vi "App - RUS scan V1.vi"(0 "Lock-in DAQ settings":T9={"Lockin mode"=enum."NI-DAQ", "DAQmx Device"="Dev2", "SR Lockin"="GPIB0::10::INSTR", "Clock Multiplier"=64, "Low-pass filter"=enum."No filtering", "Ranges and couplings "=[{"Range"=2.5, "Coupling"=10106}], "Samples per read"=20, "Record IF"=FALSE, "Auto-phase"=FALSE} {"Ranges and couplings"."Coupling" items=["default"=-1, "RSE"=10083, "NRSE"=10078, "Differential"=10106, "Pseudodifferential"=12529]}, 1 "Save data settings":T10={"Save data"=TRUE, "Data Root Path"=path "E:/data/Ultrasound/Experiment/ProbeTest/Birdcage/YBCO_6_opt/1_test", "File Prefix"="300.05900K_100_3500_2.00000V_0.65333T_Jul07-2013__19-17-53_", "File Format"=enum."BINARY", "Save column names"=FALSE, "File Comments"="\r\nColumns:Frequency\\tX\\tY\r\n    ITC Temp= 299.200000\r\n    LTC Temp= 0.000000\r\n          ITC_set=295.00000\r\n", "User/Prj"="<User Name/Project Description>"}, 5 "temperature":dbl=300.059, 7 "sweep settings":T6={"wait between \nsweeps (min) "=0.0, "Bypass error dialog"=TRUE, "time in gamma PID?"=FALSE, "power PID?"=FALSE, "range factor"=1.05, "min gamma(kHz)"=0.002, "max step(Hz)"=3000.0, "min step(Hz)"=0.002, "save freq units"=enum."kHz", "Zero amplitude\nat the end"=FALSE, "time in Gamma --OK"=FALSE, "scan mode"=enum."uniform", "power mode "=enum."power vs Temp"}, 9 "Fast swep settings":T8={"Update rate (Hz)"=500.0, "Start F, Hz"=100000.0, "Stop F"=3500000.0, "Number of points"=225000, "Amplitude"=2.0, "Init&amplitude"=TRUE, "IF"=1000.0, "Time constant"=0.001} {"IF" format="%#_6p"; "Amplitude" min=0.0 max=2.5; "Number of points" format="%.0p"; "Stop F" format="%#_6p"; "Start F, Hz" format="%#_6p"; "Update rate (Hz)" format="%0.2f"}, 11 "error in (no error)":errorcluster) -> (6 "Actual file path":path=path "E:/data/Ultrasound/Experiment/ProbeTest/Birdcage/YBCO_6_opt/1_test/July_2013/070713/300.06500K_100_3500_2.00000V_0.65334T_Jul07-2013__19-10-21_001_070713.bin", 15 "error out":errorcluster)   [LabVIEW 2012]
uses:
  RUS/Controls/Sweep settings.ctl
  File/Controls/Save data settings.ctl
  File/Controls/File formats.ctl
  RUS/Controls/Lock-in DAQ settings.ctl
  single sweep - frequency chunks.ctl
  single sweep - adaptive parameters.ctl
  next chunk -- parameters.ctl
  find peak -- parameters.ctl
  wavepacket.ctl
  adaptive sweep UI controls.ctl
  next chunk -- algorithm.ctl
  cursor action.ctl
  four-corner circle transformation.ctl
  circle corners.ctl
  next chunk -- action.ctl
  <vilib>/Utility/error.llb/DialogType.ctl
  circle center from three points.vi
  draw a line.vi
  draw a circle.vi
  generate linear region.vi
  <resource>/objmgr/daqmx.rc
panel:
  out "#data points so far":i32
  out "near gamma (kHz)":dbl
  out "near omega (kHz)":dbl
  in  "chunks":T1={"start F (Hz)"=100000.0, "stop F (Hz)"=3500000.0, "total number of points"=225000, "chunk size"=20, "freq step (Hz)"=15.11111111111111, "update rate (Hz)"=500.0, "adaptive parameters"={"peaks are known -- parameters"={"Def Gamma (kHz)"=5.0, "dV"=17.0, "time in Gamma (sec)"=4.0, "phi-star"=0.0, "all peaks (kHz)"=[579.06065, 764.63094, 998.91771, 1195.94347, 1317.30255, 1610.74434, 1757.57876, 1822.74817, 1942.37333, 2228.49853, 2291.40604, 2372.52609], "delta t (sec)"=0.002, "default step (Hz)"=95.23809523809524, "all gamma (kHz)"=[2.59786, 0.92489, 0.62142, 0.73273, 10.28068, 16.63503, 15.05454, 10.1269, 1.14235, 18.95685, 0.57285, 10.32905], "peaks OK"=TRUE, "gamma OK"=TRUE, "near omega (kHz)"=0.0, "near gamma (kHz)"=0.0, "min step (Hz)"=0.002, "max step(Hz)"=3000.0, "min gamma (kHz)"=0.002, "all time in gamma (sec)"=[], "time in gamma OK"=FALSE}, "find peak - parameters"={"wavepacket"={"R"=0.5, "wave number"=17.0, "delta k"=7.0, "radii vector"=[], "radial section"=[], "wave vector"=22.0, "wavepacket is"=TRUE}, "number of grid points"=70, "decimation threshold"=1, "Voltage range"=0.1, "target freq step"=20.0, "target spot size"=0.05, "factor"=1.0, "another factor"=1.0, "analyze last # sec"=3, "scale factor"=3}}, "total sweep time (sec)"=450.0, "chunk time (sec)"=0.04, "spot size (V)"=0.0, "uniform freq step (Hz)"=15.11111111111111, "next start freq (Hz)"=308533.3333333356} {"next start freq (Hz)" format="%#9_8f"; "uniform freq step (Hz)" format="%#_3f"; "spot size (V)" format="%#_2f"; "adaptive parameters"."find peak - parameters"."wavepacket"."delta k" format="%#_3f"; "adaptive parameters"."find peak - parameters"."wavepacket"."wave number" format="%#_3f"; "adaptive parameters"."find peak - parameters"."wavepacket"."R" format="%#_3f"; "freq step (Hz)" format="%#4_4f"; "stop F (Hz)" format="%#_3f"; "start F (Hz)" format="%#_3f"}
  in  "adaptive state":T2={"peaks are known -- parameters"={"Def Gamma (kHz)"=5.0, "dV"=17.0, "time in Gamma (sec)"=4.0, "phi-star"=0.0, "all peaks (kHz)"=[579.06065, 764.63094, 998.91771, 1195.94347, 1317.30255, 1610.74434, 1757.57876, 1822.74817, 1942.37333, 2228.49853, 2291.40604, 2372.52609], "delta t (sec)"=0.002, "default step (Hz)"=95.23809523809524, "all gamma (kHz)"=[2.59786, 0.92489, 0.62142, 0.73273, 10.28068, 16.63503, 15.05454, 10.1269, 1.14235, 18.95685, 0.57285, 10.32905], "peaks OK"=TRUE, "gamma OK"=TRUE, "near omega (kHz)"=0.0, "near gamma (kHz)"=0.0, "min step (Hz)"=0.002, "max step(Hz)"=3000.0, "min gamma (kHz)"=0.002, "all time in gamma (sec)"=[], "time in gamma OK"=FALSE}, "find peak - parameters"={"wavepacket"={"R"=0.5, "wave number"=17.0, "delta k"=7.0, "radii vector"=[], "radial section"=[], "wave vector"=22.0, "wavepacket is"=TRUE}, "number of grid points"=70, "decimation threshold"=1, "Voltage range"=0.1, "target freq step"=20.0, "target spot size"=0.05, "factor"=1.0, "another factor"=1.0, "analyze last # sec"=3, "scale factor"=3}} {"find peak - parameters"."wavepacket"."delta k" format="%#_3f"; "find peak - parameters"."wavepacket"."wave number" format="%#_3f"; "find peak - parameters"."wavepacket"."R" format="%#_3f"}
  in  "Tab : everything":enum32{"main", "everything else", "adaptive"}(tab)
  in  "complex plane scale gauge":dbl(slide)=0.006089279606872359 caption="Volts" scale=0.0001..0.1
  in  "show plot pallets":bool
  in  "highlight last # sec":dbl=5.0
  out "Plot:response":cluster{dbl[], dbl[]}[](graph)
  out "Plot:complex plane":cluster{dbl[], dbl[]}[](graph)
  in  "progress (sec)":dbl(slide)=27.441999999999098 caption="seconds" min=80.0 max=80.0 scale=0.0..42.0
  in  "Plot when running":bool
  in  "Graph update rate, ms":u32=50
  in  "stop":bool
  out "Progress, %":u8(slide) scale=0.0..100.0
  in  "Tab : sweep controls":enum32{"Main controls", "File", "Advanced"}(tab)
  in  "Manual\nPhase":dbl(slide) scale=-180.0..180.0
  out "Error status byte\n(bit 5 - FAST aborted)":u8 format="%08b"
  out "STD status byte":u8 format="%08b"
  out "DO array  making time":u32=1
  out "DO write time, ms":u32=25
  out "Loop counter":i32=11249
  out "Pre-sweep delay, s":dbl=0.2
  out "Samples in buffer":u32
  out "Actual setup time, ms":u32=1795
  out "line two":cluster{dbl[], dbl[]}
  out "circle":cluster{dbl[], dbl[]}
  out "line one":cluster{dbl[], dbl[]}
  out "frequency":dbl[](array[numeric])
  out "complex data":cdb[](array[numeric])
  out "fancy circles":cluster{dbl[], dbl[]}[](array[cluster])
  out "fancy lines":cluster{dbl[], dbl[]}[](array[cluster])=[{[579.06065, 579.06065], [-0.001, 0.001]}, {[764.63094, 764.63094], [-0.001, 0.001]}, {[998.91771, 998.91771], [-0.001, 0.001]}, {[1195.94347, 1195.94347], [-0.001, 0.001]}, {[1317.30255, 1317.30255], [-0.001, 0.001]}, {[1610.74434, 1610.74434], [-0.001, 0.001]}, {[1757.57876, 1757.57876], [-0.001, 0.001]}, {[1822.74817, 1822.74817], [-0.001, 0.001]}, {[1942.37333, 1942.37333], [-0.001, 0.001]}, {[2228.49853, 2228.49853], [-0.001, 0.001]}, {[2291.40604, 2291.40604], [-0.001, 0.001]}, {[2372.52609, 2372.52609], [-0.001, 0.001]}]
  # "SRS Lockin related"
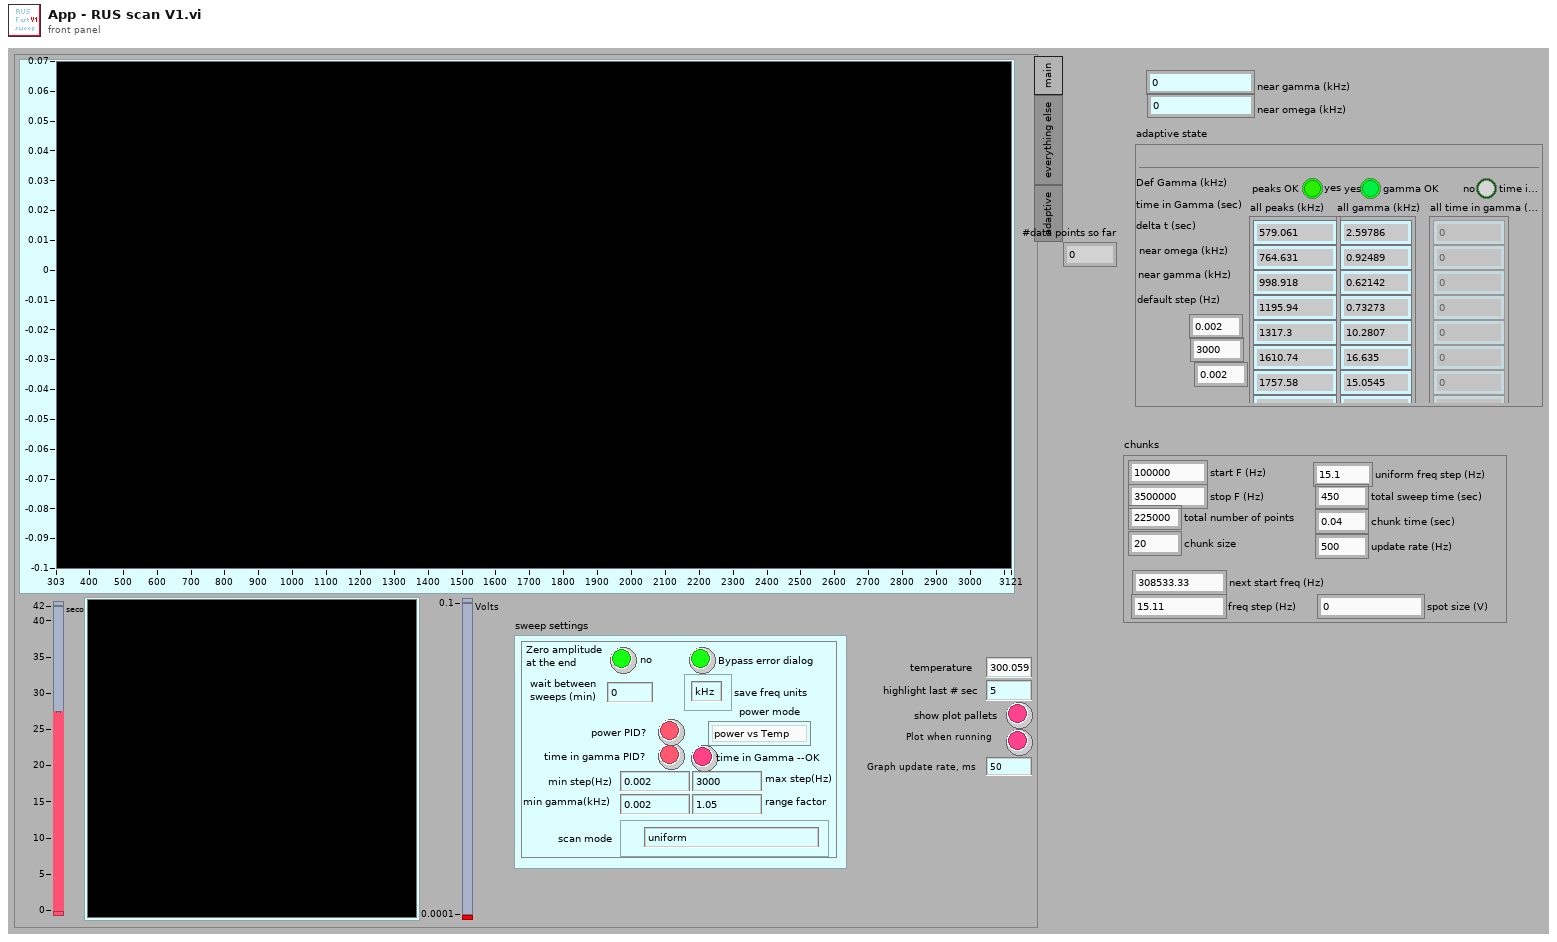
[diagram p1: front panel]
types:
  T1 = typedef "single sweep - frequency chunks.ctl" = cluster{"start F (Hz)":dbl, "stop F (Hz)":dbl, "total number of points":i32, "chunk size":i32, "freq step (Hz)":dbl, "update rate (Hz)":dbl, "adaptive parameters":T2, "total sweep time (sec)":dbl, "chunk time (sec)":dbl, "spot size (V)":dbl, "uniform freq step (Hz)":dbl, "next start freq (Hz)":dbl}
  T2 = typedef "single sweep - adaptive parameters.ctl" = cluster{"peaks are known -- parameters":T3, "find peak - parameters":T4}
  T3 = typedef "next chunk -- parameters.ctl" = cluster{"Def Gamma (kHz)":dbl, "dV":dbl, "time in Gamma (sec)":dbl, "phi-star":dbl, "all peaks (kHz)":dbl[], "delta t (sec)":dbl, "default step (Hz)":dbl, "all gamma (kHz)":dbl[], "peaks OK":bool, "gamma OK":bool, "near omega (kHz)":dbl, "near gamma (kHz)":dbl, "min step (Hz)":dbl, "max step(Hz)":dbl, "min gamma (kHz)":dbl, "all time in gamma (sec)":dbl[], "time in gamma OK":bool}
  T4 = typedef "find peak -- parameters.ctl" = cluster{"wavepacket":T5, "number of grid points":i32, "decimation threshold":i32, "Voltage range":dbl, "target freq step":dbl, "target spot size":dbl, "factor":dbl, "another factor":dbl, "analyze last # sec":i32, "scale factor":i32}
  T5 = typedef "wavepacket.ctl" = cluster{"R":dbl, "wave number":dbl, "delta k":dbl, "radii vector":dbl[], "radial section":cdb[], "wave vector":dbl, "wavepacket is":bool}
  T6 = typedef "adaptive sweep UI controls.ctl" = cluster{"wait between \nsweeps (min) ":dbl, "Bypass error dialog":bool, "time in gamma PID?":bool, "power PID?":bool, "range factor":dbl, "min gamma(kHz)":dbl, "max step(Hz)":dbl, "min step(Hz)":dbl, "save freq units":enum16{"kHz", "Hz"}, "Zero amplitude\nat the end":bool, "time in Gamma --OK":bool, "scan mode":T7, "power mode ":enum16{"power vs Temp", "power vs Time"}}
  T7 = typedef "next chunk -- algorithm.ctl" = enum16{"peak position is known", "uniform", "predictive", ""}
  T8 = typedef "Sweep settings.ctl" = cluster{"Update rate (Hz)":dbl, "Start F, Hz":dbl, "Stop F":dbl, "Number of points":i32, "Amplitude":dbl, "Init&amplitude":bool, "IF":dbl, "Time constant":dbl}
  T9 = typedef "Lock-in DAQ settings.ctl" = cluster{"Lockin mode":enum16{"SRS", "NI-DAQ"}, "DAQmx Device":tag, "SR Lockin":refnum<visa-resource-name>, "Clock Multiplier":i32, "Low-pass filter":enum16{"No filtering", "Butterworth", "Bessel"}, "Ranges and couplings ":cluster{"Range":dbl, "Coupling":i32}[], "Samples per read":i32, "Record IF":bool, "Auto-phase":bool}
  T10 = typedef "Save data settings.ctl" = cluster{"Save data":bool, "Data Root Path":path, "File Prefix":string, "File Format":T11, "Save column names":bool, "File Comments":string, "User/Prj":string}
  T11 = typedef "File formats.ctl" = enum16{"TDMS", "ASCII", "BINARY"}
  T12 = typedef "RUS settings.ctl" = cluster{"NI-DAQ lockin settings":T13, "Fast swep settings":T8, "Pre-sweep delay, s":dbl, "Lockin mode":enum16{"SRS", "NI-DAQ"}, "SR Lockin":refnum<visa-resource-name>, "DAQmx Device":tag, "Clock Multiplier":i32, "Fast Sweep Data Out":cluster{"DO clock task":refnum<k21>, "DO task":refnum<k21>, "Update clock task":refnum<k21>, "DAQ lockin task":refnum<k21>, "Pre-sweep counter task":refnum<k21>}, "Lockin Range, V":sgl, "F Array":dbl[], "Freq. update clock terminal":string, "DO Clock Rate (Hz)":dbl, "ADC clock terminal":string, "Pre-sweep counter terminal":string, "Samples per read":i32, "DO clock terminal":string, "Pre-sweep points":i32, "F points per write":i32, "Total sweep time, s":dbl, "Initial SYNTH phase":dbl, "Record IF":bool, "Save data settings":T10, "Data file path":path, "New data user event":refnum<user-event>, "Stop user event":refnum<user-event>, "Number of channels":i32, "Auto-phase":bool}
  T13 = typedef "RUS NI-DAQ Lockin Settings.ctl" = cluster{"Samples per sine wave":i32, "Sine waves per freq step":i32, "Output Representation":enum16{"Real/Imaginary", "Polar"}, "Low-pass filter":enum16{"No filtering", "Butterworth", "Bessel"}, "Ranges and couplings ":cluster{"Range":dbl, "Coupling":i32}[]}
  T14 = typedef "next chunk -- action.ctl" = enum16{"empty", "init - uniform", "next chunk - uniform", "next chunk - peaks are known", "init - peaks are known", ""}
  T15 = typedef "circle corners.ctl" = cluster{"z (-pi/2)":cdb, "z(inf)":cdb, "z (pi/2)":cdb, "z center":cdb, "z(0)":cdb, "radius":dbl}
  T16 = typedef "four-corner circle transformation.ctl" = enum16{"z(c) z(inf)", "z(c) z(zero)", "fix phase", "calculate lorentzian", "z(0) z(+-pi/2)", "shift to zcenter"}
  T17 = typedef "cursor action.ctl" = enum16{"range", "read", "write", "check", "zoom out"}
  T18 = typedef "DialogType.ctl" = u16
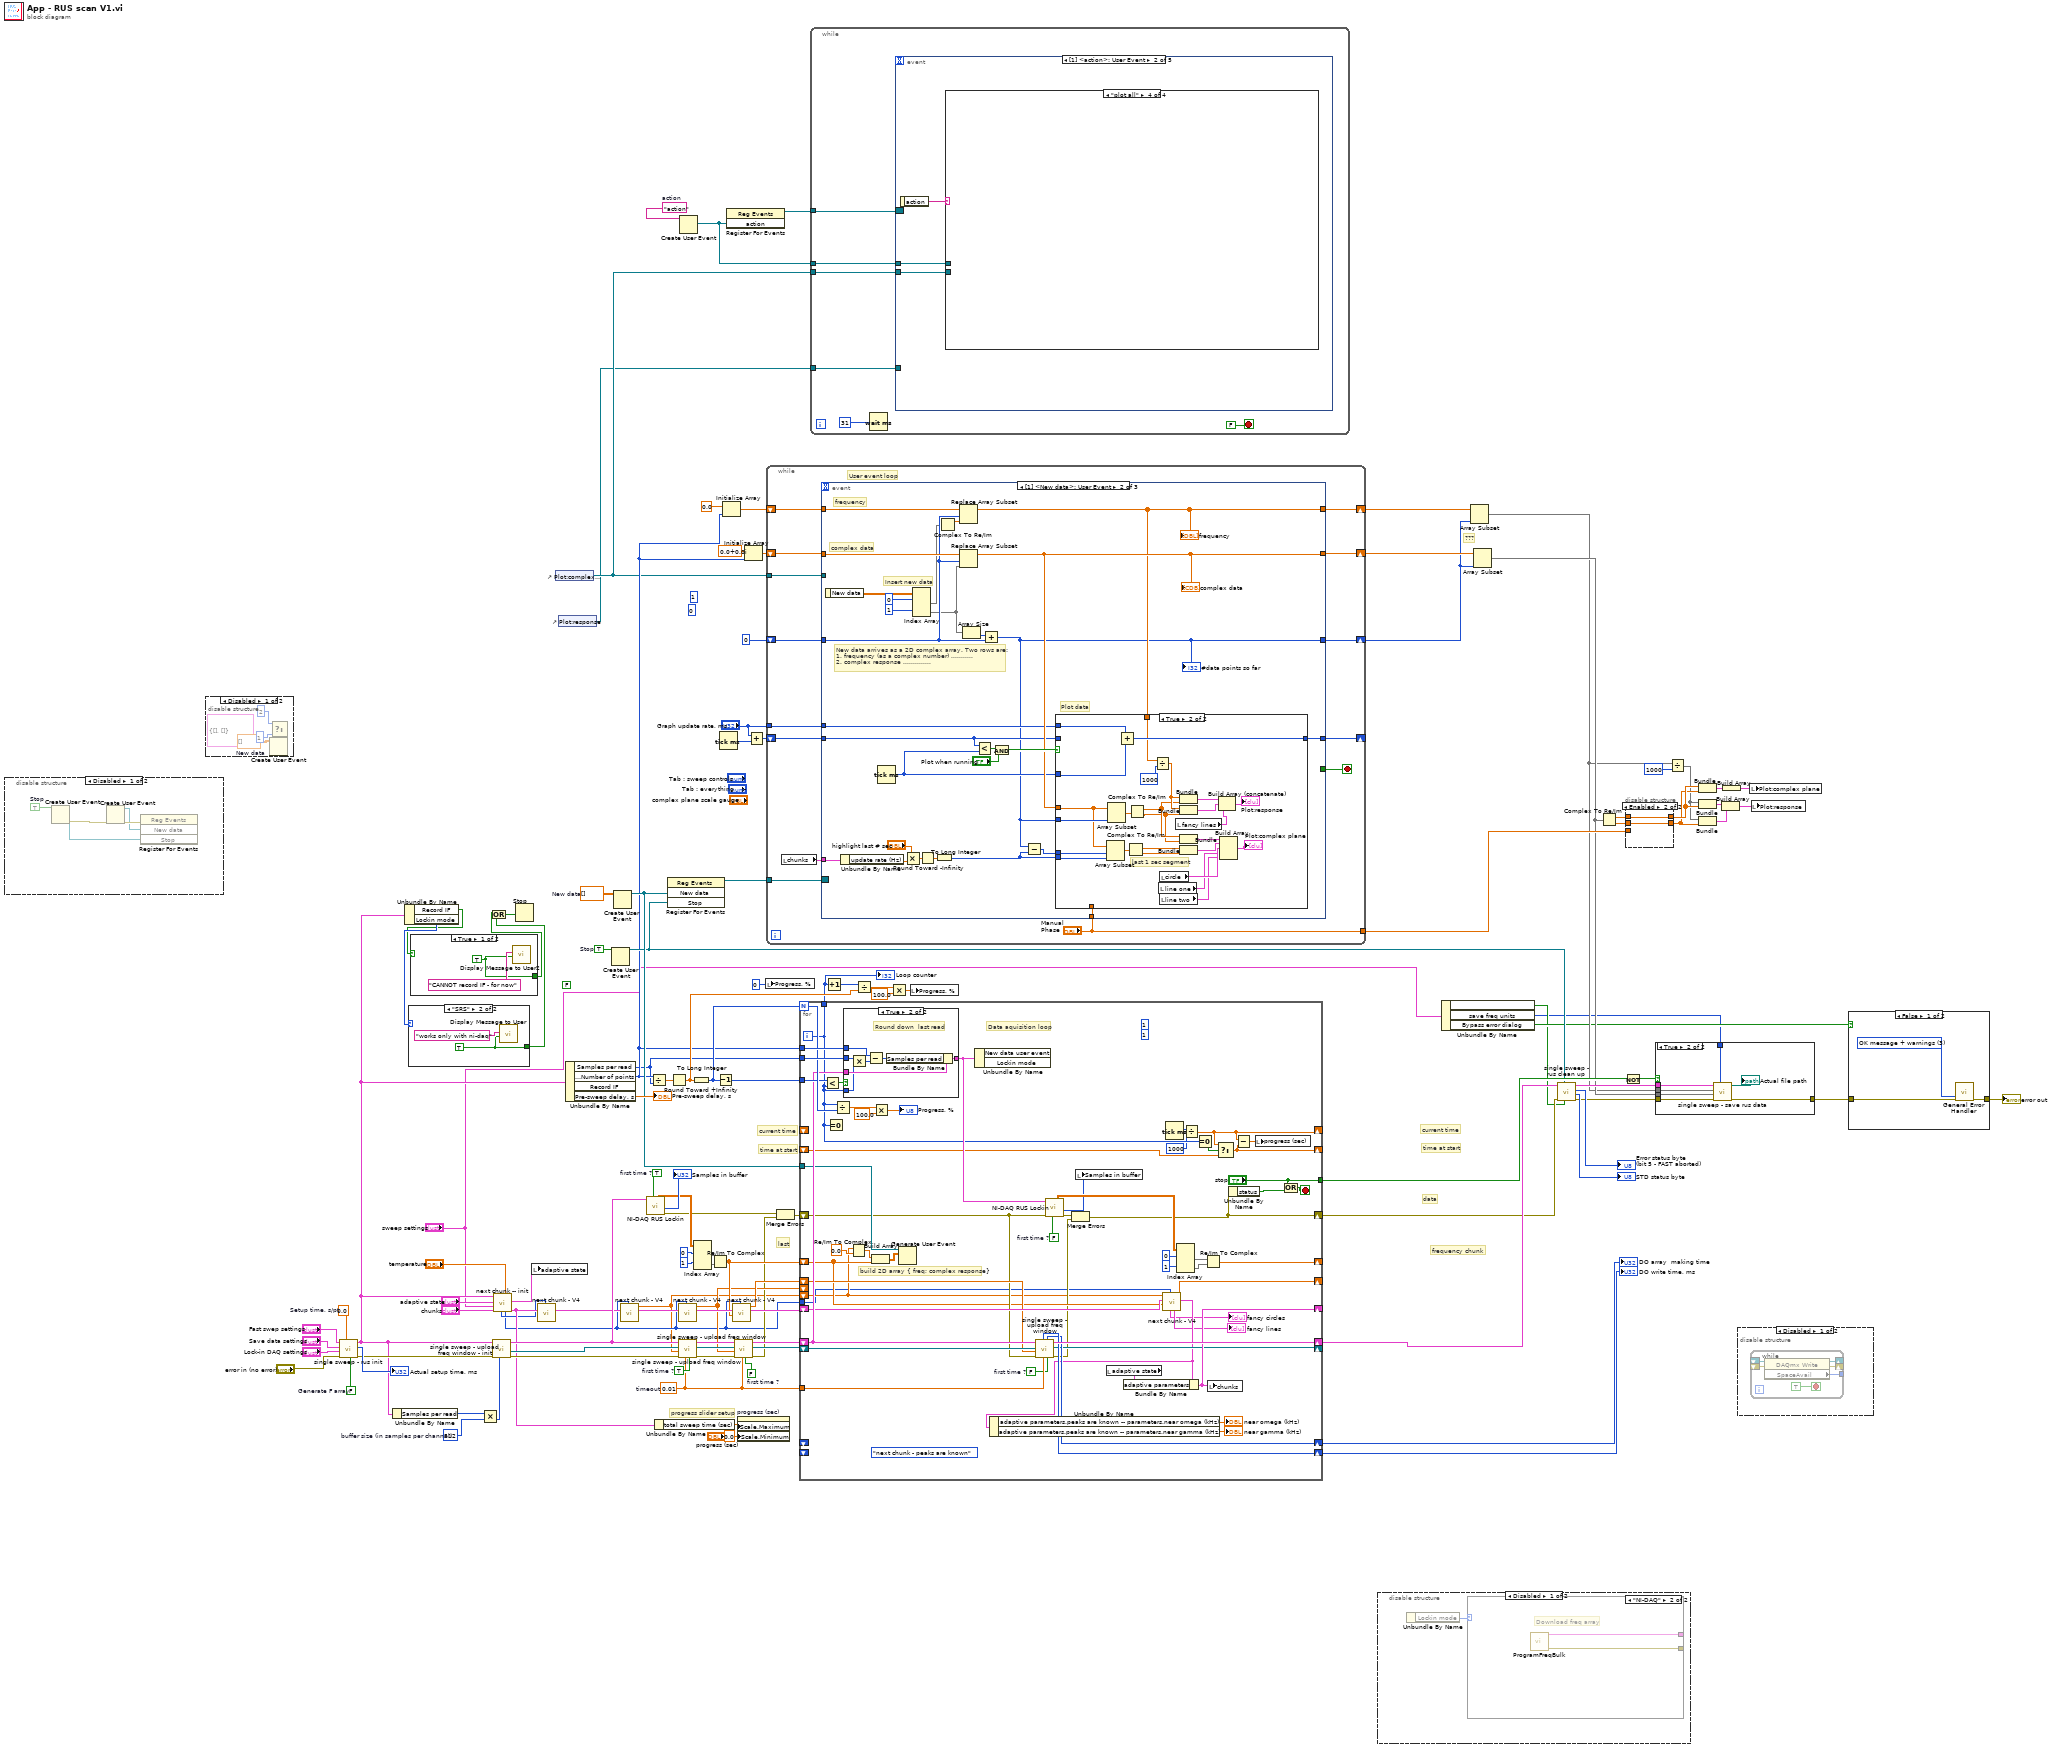
[diagram p0: block diagram]
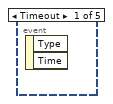
[diagram p2: hidden frame]
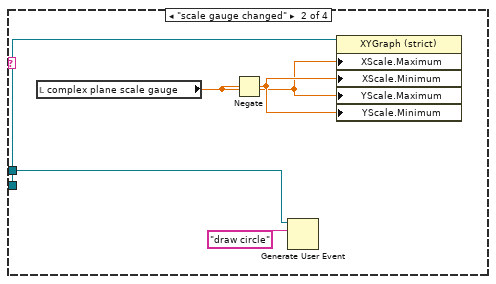
[diagram p4: hidden frame]
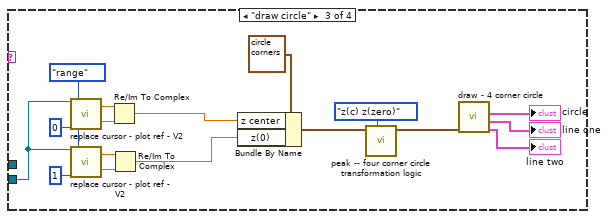
[diagram p5: hidden frame]
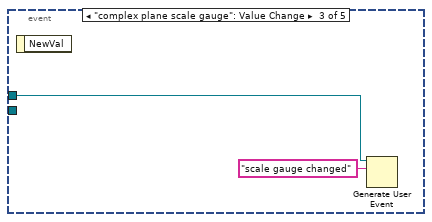
[diagram p6: hidden frame]
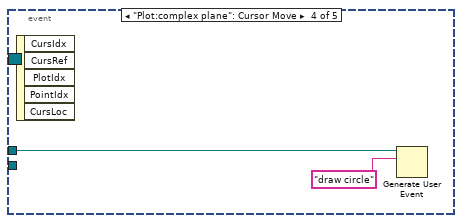
[diagram p7: hidden frame]
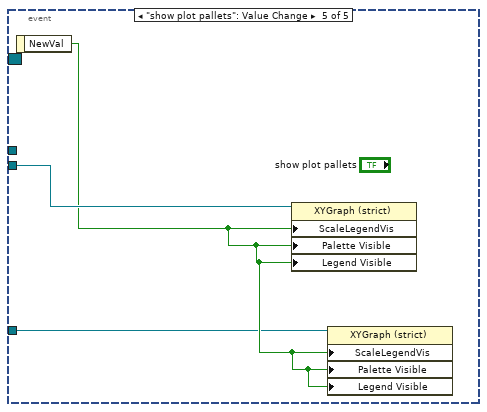
[diagram p8: hidden frame]
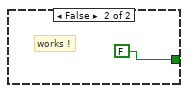
[diagram p10: hidden frame]
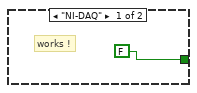
[diagram p13: hidden frame]
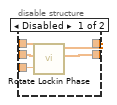
[diagram p17: hidden frame]
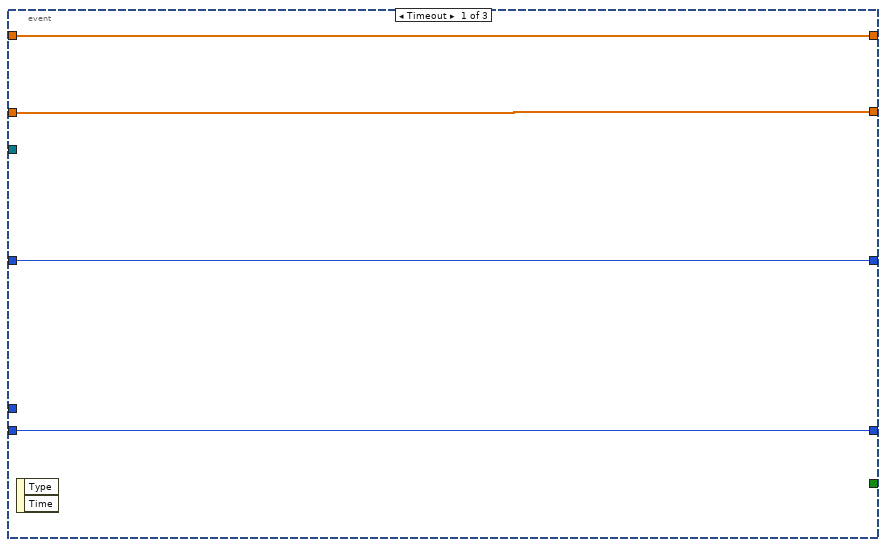
[diagram p18: hidden frame]
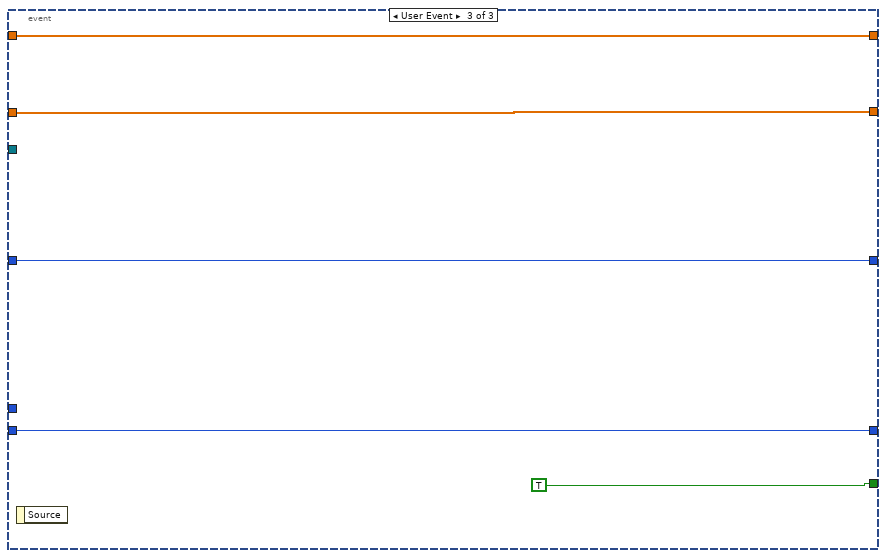
[diagram p20: hidden frame]
diagram:
  w5 = "action"  # action
  w28 = TRUE  # first time ?
  w29 = FALSE  # Generate F array
  w30 = 0.0  # Setup time, s/pt
  w33 = u32 512  # buffer size (in samples per channel)
  w48 = FALSE  # first time ?
  (unwired) 0 ("disabled index (col)")
  (unwired) FALSE
  (unwired) 1 ("dimension size")
  w76 = cdb[][] []  # New data
  w78 = TRUE  # Stop
  w82 = TRUE  # first time ?
  w41 = 0.01  # timeout
  # "data"
  # "frequency chunk"
  # "last"
  # "time at start"
  # "current time"
  # "time at start"
  # "current time"
  # "progress slider setup"
  # "???"
  n1 = disable-structure shown="Disabled" {
    frame Disabled {
      w124 = TRUE  # Stop
      n2 = Create User Event(user event datatype=w124) -> (user event=w121:refnum<user-event>, error out=w123:errorcluster)  [unwired: 1 in]
      n3 = Create User Event(error in=w123) -> (user event datatype=w119:cluster{}, user event=w120:refnum<user-event>, error out=w122:errorcluster)
      n4 = register-events(error in=w122, w120, w121) -> ()  [unwired: 1 in, 2 out]
    }
    frame Enabled {
    }
  }
  n5 = disable-structure shown="Disabled" {
    frame Disabled {
      w125 = cdb[][] []  # New data
      (unwired) cluster{cdb[], dbl[]} {[], []} ("Newer data")
      n6 = Create User Event(user event datatype=w125) -> ()  [unwired: 1 in, 2 out]
      n7 = Select(t=2 ("dimension size"), f=1 ("dimension size")) -> ()  [unwired: 1 in, 1 out]
    }
    frame Enabled {
    }
  }
  n8 = call "single sweep - rus init.vi"("Generate F array"=w29, "Setup time, s/pt"=w30, "error in (no error)"="error in (no error)", "Lock-in DAQ settings"="Lock-in DAQ settings", "Save data settings"="Save data settings", "Fast swep settings"="Fast swep settings") -> ("error out"=w85:errorcluster, "Actual setup time, ms"=→"Actual setup time, ms":u32, "RUS settings out"=w18:T12)  [unwired: 2 in, 1 out]
  n9 = Unbundle By Name(w18) -> ("Samples per read"=w31:i32)
  n10 = Unbundle By Name(w18) -> ("Record IF"=w58:bool, "Lockin mode"=w84:enum16{"SRS", "NI-DAQ"})
  n11 = case shown="\"SRS\"" w84 {
    tunnel: [FALSE w129] -> w60
    frame "NI-DAQ" {
      # "works !"
    }
    frame "SRS" {
      w129 = TRUE
      n12 = call "Display Message to User"("Enable"=w129, "Message"="works only with ni-daq") -> ()  [unwired: 8 in, 2 out]
    }
  }
  n13 = case shown="True" w58 {
    tunnel: [w131 FALSE] -> w59
    frame True {
      w131 = TRUE
      n14 = call "Display Message to User2"("Enable"=w131, "Message"="CANNOT record IF - for now") -> ()  [unwired: 8 in, 2 out]
    }
    frame False {
      # "works !"
    }
  }
  n15 = Multiply(x=w31, y=w33) -> (x*y=w32:u32)
  n16 = Or(x=w59, y=w60) -> (x .or. y?=w57:bool)
  n17 = call "single sweep - upload freq window - init.vi"("buffer size (in samples per channel)"=w32, "error in (no error)"=w85, "RUS settings"=w18) -> ("error - out"=w37:errorcluster, "task out"=w83:refnum<k21>, "RUS settings out"=w49:T12)  [unwired: 6 in]
  n18 = call "next chunk -- init.vi"("temperature"="temperature", "chunks"="chunks", "sweep settings"="sweep settings", "adaptive parameters"="adaptive state", "RUS settings"=w18) -> ("chunks out"=w17:T1, "adaptive parameters out"=w15:T2, "next chunk action"=w11:T14, "next chunk init action"=w14:T14)  [unwired: 3 in]
  n19 = Stop(stop? (T)=w57) -> ()
  n20 = local write "adaptive state"(w15) -> ()
  n21 = call "next chunk - V4.vi"("next chunk action"=w14, "chunks"=w17) -> ("chunks out"=w12:T1)  [unwired: 6 in, 3 out]
  n22 = control-ref of="Plot:complex plane"() -> (w3:refnum<vi>)
  n23 = control-ref of="Plot:response"() -> (w1:refnum<vi>)
  n24 = Unbundle By Name(w18) -> ("Samples per read"=w50:i32, "Fast swep settings.Number of points"=w51:i32, "Pre-sweep delay, s"=→"Pre-sweep delay, s":dbl)  [unwired: 1 out]
  n25 = Create User Event(user event datatype=w78) -> (user event=w64:refnum<user-event>)  [unwired: 1 in, 1 out]
  n26 = Create User Event(user event datatype=w76) -> (user event=w77:refnum<user-event>)  [unwired: 1 in, 1 out]
  n27 = call "next chunk - V4.vi"("next chunk action"=w11, "chunks"=w12) -> ("F Array out"=w10:dbl[])  [unwired: 6 in, 3 out]
  n28 = call "NI-DAQ RUS Lockin.vi"("Init?"=w28, "RUS settings"=w49) -> ("error out"=w21:errorcluster, "AvailSampPerChan"=→"Samples in buffer":u32, "Lockin out"=w22:dbl[][])  [unwired: 6 in, 1 out]
  n29 = Divide(x=w51, y=w50) -> (x/y=w116:dbl)
  n30 = Unbundle By Name(w17) -> ("total sweep time (sec)"=w56:dbl)
  n31 = register-events(w77, w64) -> (reference out=w79:refnum<event-registration>)  [unwired: 2 in, 1 out]
  n32 = Round Toward +Infinity(x=w116) -> (ceil(x): smallest int >= x=w110:dbl)
  n33 = call "single sweep - upload freq window.vi"("first time ?"=w82, "timeout"=w41, "error in (no error)"=w37, "F-window array"=w10, "task in"=w83, "RUS settings"=w49) -> ("error out"=w36:errorcluster, "task out"=w44:refnum<k21>, "RUS settings out"=w47:T12)  [unwired: 1 in, 2 out]
  n34 = call "next chunk - V4.vi"("next chunk action"=w11, "chunks"=w12) -> ("chunks out"=w43:T1, "F Array out"=w34:dbl[])  [unwired: 6 in, 2 out]
  n35 = Create User Event(user event datatype=w5) -> (user event=w2:refnum<user-event>)  [unwired: 1 in, 1 out]
  n36 = To Long Integer(number=w110) -> (32bit integer=w94:i32)
  n37 = Index Array(array=w22, index (row) #1=0 ("index"), index (row) #2=1 ("length")) -> (element #1=w24:dbl[], element #2=w23:dbl[])  [unwired: 2 in]
  n38 = Re/Im To Complex(1:w23, 2:w24) -> (0:w35:cdb[])
  n39 = Decrement(x=w94) -> (x-1=w106:i32)
  n40 = Tick Count (ms)() -> (millisecond timer value=w117:u32)
  n41 = Initialize Array(0.0 ("Numeric"), w51) -> (w73:dbl[])
  n42 = register-events(w2) -> (reference out=w4:refnum<event-registration>)  [unwired: 2 in, 1 out]
  n43 = call "next chunk - V4.vi"("next chunk action"=w11, "x + iy"=w35, "chunks"=w43) -> ("chunks out"=w42:T1, "F Array out"=w39:dbl[])  [unwired: 5 in, 2 out]
  n44 = call "single sweep - upload freq window.vi"("first time ?"=w48, "timeout"=w41, "error in (no error)"=w36, "F-window array"=w34, "task in"=w44, "RUS settings"=w47) -> ("error out"=w20:errorcluster, "task out"=w45:refnum<k21>, "RUS settings out"=w46:T12)  [unwired: 1 in, 2 out]
  n45 = property on="progress (sec)" class="Slide (strict)"("Scale.Maximum"=w56, "Scale.Minimum"=0.0 ("Data Entry Limits:Minimum")) -> ()  [unwired: 2 in, 2 out]
  n46 = Initialize Array(cdb 0.0+0.0i ("Numeric"), w51) -> (w108:cdb[])
  n47 = Add(x="Graph update rate, ms", y=w117) -> (x+y=w87:u32)
  n48 = local write "Progress, %"(u8 0 ("Progress")) -> ()
  n49 = while {
    tunnel: w79 -> [w147]
    shift-right: [w145] -> w101
    shift-left: w108 -> [w144]
    shift-right: [w141] -> _
    shift-left: w87 -> [w143]
    tunnel: "Graph update rate, ms" -> [w142]
    shift-right: [w139] -> w61
    shift-left: 0 ("disabled index (col)") -> [w140]
    tunnel: ["Manual\nPhase"] -> w98
    shift-right: [w136] -> w62
    shift-left: w73 -> [w138]
    tunnel: w3 -> [w134]
    stop <- w146 stop-if-true
    # "User event loop"
    n50 = local read "chunks"() -> (w135:T1)
    n51 = event shown="[1] <New data>: User Event" {
      selector: w147 -> [_ _ _]
      dyn-events: _ -> [_ _ _]
      timeout: _ -> [_ _ _]
      tunnel: [_ _ TRUE] -> w146
      tunnel: [w151 w176 w210] -> w145
      tunnel: w144 -> [w151 w177 w210]
      tunnel: w143 -> [w150 w172 w209]
      tunnel: w142 -> [_ w170 _]
      tunnel: [w150 w179 w209] -> w141
      tunnel: w140 -> [w149 w164 w208]
      tunnel: [w149 w157 w208] -> w139
      tunnel: w138 -> [w148 w166 w207]
      tunnel: "Manual\nPhase" -> [_ w175 _]
      tunnel: [w148 w165 w207] -> w136
      tunnel: w135 -> [_ w160 _]
      tunnel: w134 -> [_ _ _]
      event Timeout {
        n52 = event-data() -> ()  [unwired: 3 out]
      }
      event User Event {
        # "complex data"
        # "frequency"
        # "Plot data"
        # "New data arrives as a 2D complex array. Two rows are: \n1. frequency (as a complex number) ........... \n2. complex response .............."
        # "Insert new data"
        n53 = event-data() -> ("New data"=w169:cdb[][])  [unwired: 1 out]
        n54 = Unbundle By Name(w160) -> ("update rate (Hz)"=w159:dbl)
        n55 = Tick Count (ms)() -> (millisecond timer value=w171:u32)
        n56 = Multiply(x="highlight last # sec", y=w159) -> (x*y=w158:dbl)
        n57 = Index Array(array=w169, index (row) #1=0 ("disabled index (col)"), index (row) #2=1 ("disabled index (col)")) -> (element #1=w163:cdb[], element #2=w155:cdb[])  [unwired: 2 in]
        n58 = Round Toward -Infinity(1:w158) -> (0:w153:dbl)
        n59 = To Long Integer(number=w153) -> (32bit integer=w152:i32)
        n60 = Complex To Re/Im(x + iy=w163) -> (x=w162:dbl[])  [unwired: 1 out]
        n61 = Replace Array Subset(array=w166, new element=w162, index=w164) -> (w165:dbl[])
        "frequency" <- w165
        n62 = Replace Array Subset(array=w177, new element=w155, index=w164) -> (w176:cdb[])
        "complex data" <- w176
        n63 = Array Size(array=w155) -> (size(s)=w154:i32)
        n64 = Less?(x=w172, y=w171) -> (x < y?=w174:bool)
        n65 = Add(x=w154, y=w164) -> (x+y=w157:i32)
        "#data points so far" <- w157
        n66 = And(x=w174, y="Plot when running") -> (x .and. y?=w178:bool)
        n67 = Subtract(x=w157, y=w152) -> (x-y=w156:i32)
        n68 = case shown="True" w178 {
          tunnel: w176 -> [_ w193]
          tunnel: w171 -> [_ w202]
          tunnel: [w180 w201] -> w179
          tunnel: w172 -> [w180 _]
          tunnel: w165 -> [_ w189]
          tunnel: w157 -> [_ w199]
          tunnel: w175 -> [_ _]
          tunnel: w170 -> [_ w203]
          tunnel: w156 -> [_ w195]
          tunnel: w152 -> [_ w194]
          frame False {
          }
          frame True {
            # "last 1 sec segment"
            n69 = Array Subset(array=w193, index=w195, length=w194) -> (w196:cdb[])
            n70 = Array Subset(array=w193, length=w199) -> (w198:cdb[])  [unwired: 1 in]
            n71 = Add(x=w203, y=w202) -> (x+y=w201:u32)
            n72 = Complex To Re/Im(x + iy=w196) -> (x=w192:dbl[], y=w191:dbl[])
            n73 = Complex To Re/Im(x + iy=w198) -> (x=w186:dbl[], y=w185:dbl[])
            n74 = Divide(x=w189, y=1000 ("dimension size")) -> (x/y=w188:dbl[])
            n75 = local read "line one"() -> (w182:cluster{dbl[], dbl[]})
            n76 = local read "circle"() -> (w183:cluster{dbl[], dbl[]})
            n77 = local read "line two"() -> (w181:cluster{dbl[], dbl[]})
            n78 = local read "fancy lines"() -> (w184:cluster{dbl[], dbl[]}[])
            n79 = Bundle(w188, w186) -> (w206:cluster{dbl[], dbl[]})  [unwired: 1 out]
            n80 = Bundle(w188, w185) -> (w204:cluster{dbl[], dbl[]})  [unwired: 1 out]
            n81 = Bundle(w186, w185) -> (w197:cluster{dbl[], dbl[]})  [unwired: 1 out]
            n82 = Bundle(w192, w191) -> (w190:cluster{dbl[], dbl[]})  [unwired: 1 out]
            n83 = Build Array (concatenate)(w206, w204, w184) -> (→"Plot:response":cluster{dbl[], dbl[]}[])
            n84 = Build Array(w197, w190, w183, w182, w181) -> (→"Plot:complex plane":cluster{dbl[], dbl[]}[])
          }
        }
      }
      event User Event {
        n85 = event-data() -> ()  [unwired: 2 out]
      }
    }
  }
  n86 = Merge Errors(w21, w20) -> (w40:errorcluster)
  n87 = for {
    N: w94 -> [w263]
    tunnel: w50 -> [w265]
    tunnel: [w235] -> w109
    tunnel: w106 -> [w259]
    tunnel: w51 -> [w266]
    tunnel: ["stop"] -> w100
    shift-right: [w254] -> w63
    shift-left: w46 -> [w256]
    tunnel: w41 -> [w255]
    shift-right: [w249] -> w81
    shift-left: _ -> [_]
    shift-right: [w220] -> _
    shift-left: w45 -> [w251]
    shift-right: [w223] -> w38
    shift-left: w40 -> [w224]
    shift-right: [w253] -> _
    shift-left: w39 -> [w225]
    shift-right: [w238] -> _
    shift-left: w42 -> [w252]
    shift-right: [w250] -> w80
    shift-left: _ -> [_]
    tunnel: w77 -> [w247]
    shift-right: [w230] -> _
    shift-left: _ -> [_]
    shift-right: [w229] -> _
    shift-left: _ -> [w231]
    shift-right: [w226] -> _
    shift-left: w35 -> [w222]
    shift-left: w34 -> [_]
    shift-left: w10 -> [w218]
    tunnel: w11 -> [w217]
    i -> [w235]
    stop <- w268 stop-if-true
    (unwired) next_chunk_--_action."next chunk - peaks are known" ("next chunk action")
    w227 = FALSE  # first time ?
    (unwired) 1 ("length")
    (unwired) 1 ("index")
    w248 = FALSE  # first time ?
    # "build 2D array { freq; complex response}"
    # "Data aquisition loop"
    n88 = Less?(x=w259, y=w235) -> (x < y?=w267:bool)
    n89 = Equal To 0?(x=w235) -> ()  [unwired: 1 out]
    n90 = Divide(x=w235, y=w263) -> (x/y=w262:dbl)
    n91 = case shown="True" w267 {
      tunnel: w266 -> [_ w276]
      tunnel: w265 -> [_ w271]
      tunnel: w235 -> [_ w270]
      tunnel: w256 -> [w269 w274]
      tunnel: [w269 w272] -> w264
      frame False {
      }
      frame True {
        # "Round down  last read"
        n92 = Multiply(x=w271, y=w270) -> (x*y=w275:i32)
        n93 = Subtract(x=w276, y=w275) -> (x-y=w273:i32)
        n94 = Bundle By Name(cluster=w274, "Samples per read"=w273) -> (w272:T12)
      }
    }
    n95 = Re/Im To Complex(1:0.0, 2:w218) -> (0:w240:cdb[])
    n96 = Build Array(w240, w222) -> (w239:cdb[][])
    n97 = Multiply(x=w262, y=100.0) -> (x*y=→"Progress, %":dbl)
    n98 = Generate User Event(user event=w247, event data cluster=w239) -> ()  [unwired: 1 in, 2 out]
    n99 = Unbundle By Name(w264) -> ()  [unwired: 2 out]
    n100 = call "single sweep - upload freq window.vi"("first time ?"=w248, "timeout"=w255, "error in (no error)"=w224, "F-window array"=w225, "task in"=w251, "RUS settings"=w256) -> ("error out"=w219:errorcluster, "task out"=w220:refnum<k21>, "RUS settings out"=w254:T12, "DO array  making time"=w249:u32, "DO write time"=w250:u32)  [unwired: 1 in]
    n101 = call "NI-DAQ RUS Lockin.vi"("Init?"=w227, "error in (no error)"=w224, "RUS settings"=w264) -> ("error out"=w221:errorcluster, "AvailSampPerChan"=w228:u32, "Lockin out"=w246:dbl[][])  [unwired: 5 in, 1 out]
    n102 = Merge Errors(w221, w219) -> (w223:errorcluster)
    n103 = local write "Samples in buffer"(w228) -> ()
    n104 = local read "adaptive state"() -> (w237:T2)
    n105 = call "next chunk - V4.vi"("next chunk action"=w217, "x + iy"=w222, "chunks"=w252, "F Array in"=w218) -> ("chunks out"=w214:T1, "F Array out"=w253:dbl[], "fancy lines"=→"fancy lines":cluster{dbl[], dbl[]}[], "fancy circles"=→"fancy circles":cluster{dbl[], dbl[]}[])  [unwired: 4 in]
    n106 = Unbundle By Name(w214) -> ("adaptive parameters.peaks are known -- parameters.near omega (kHz)"=→"near omega (kHz)":dbl, "adaptive parameters.peaks are known -- parameters.near gamma (kHz)"=→"near gamma (kHz)":dbl)
    n107 = Bundle By Name(cluster=w214, "adaptive parameters"=w237) -> (w238:T1)
    n108 = Tick Count (ms)() -> (millisecond timer value=w234:u32)
    n109 = Index Array(array=w246, index (row) #1=0 ("index"), index (row) #2=1 ("length")) -> (element #1=w243:dbl[], element #2=w242:dbl[])  [unwired: 2 in]
    n110 = Divide(x=w234, y=u32 1000) -> (x/y=w230:dbl)
    n111 = Equal To 0?(x=w235) -> (x = 0?=w232:bool)
    n112 = Re/Im To Complex(1:w242, 2:w243) -> (0:w226:cdb[])
    n113 = local write "chunks"(w238) -> ()
    n114 = Select(t=w230, s=w232, f=w231) -> (s? t:f=w229:dbl)
    n115 = Unbundle By Name(w223) -> ("status"=w257:bool)
    n116 = Subtract(x=w230, y=w229) -> (x-y=w236:dbl)
    n117 = local write "progress (sec)"(w236) -> ()
    n118 = Compound Arithmetic op=OR("stop", w257) -> (w268:bool)
  }
  "Loop counter" <- w109
  "DO array  making time" <- w81
  "DO write time, ms" <- w80
  n119 = while {
    tunnel: w4 -> [w281]
    tunnel: w3 -> [w280]
    tunnel: w2 -> [w279]
    tunnel: w1 -> [w278]
    stop <- FALSE stop-if-true
    n120 = Wait (ms)(milliseconds to wait=u32 31) -> ()  [unwired: 1 out]
    n121 = event shown="[1] <action>: User Event" {
      selector: w281 -> [_ _ _ _ _]
      dyn-events: _ -> [_ _ _ _ _]
      timeout: _ -> [_ _ _ _ _]
      tunnel: w280 -> [_ w284 _ _ w314]
      tunnel: w279 -> [_ w283 w308 w310 _]
      tunnel: w278 -> [_ _ _ _ w312]
      event Timeout {
        n122 = event-data() -> ()  [unwired: 1 in, 2 out]
      }
      event User Event {
        n123 = event-data() -> ("action"=w285:string)  [unwired: 1 in]
        n124 = case shown="\"plot all\"" w285 {
          tunnel: w284 -> [_ w288 w293 _]
          tunnel: w283 -> [_ w286 _ _]
          frame "False", Default {
          }
          frame "scale gauge changed" {
            n125 = local read "complex plane scale gauge"() -> (w289:dbl)
            n126 = Negate(x=w289) -> (-x=w290:dbl)
            n127 = Generate User Event(user event=w286, event data cluster="draw circle" ("event data")) -> ()  [unwired: 1 in, 2 out]
            n128 = property on="Property Node" class="XYGraph (strict)"(reference=w288, "XScale.Maximum"=w289, "XScale.Minimum"=w290, "YScale.Maximum"=w289, "YScale.Minimum"=w290) -> ()  [unwired: 1 in, 2 out]
          }
          frame "draw circle" {
            w305 = cursor_action."range" ("cursor action")
            n129 = call "replace cursor - plot ref - V2.vi"("Plot ref in"=w293, "cursor index"=0, "cursor action"=w305) -> ("read X"=w303:dbl, "read Y"=w302:dbl)  [unwired: 14 in, 1 out]
            n130 = call "replace cursor - plot ref - V2.vi"("Plot ref in"=w293, "cursor index"=1, "cursor action"=w305) -> ("read X"=w300:dbl, "read Y"=w299:dbl)  [unwired: 14 in, 1 out]
            n131 = Re/Im To Complex(1:w302, 2:w303) -> (0:w301:cdb)
            n132 = Re/Im To Complex(1:w299, 2:w300) -> (0:w298:cdb)
            n133 = Bundle By Name(cluster=T15 {"z (-pi/2)"=-1.0311345636926572+0.5736824521422934i, "z(inf)"=-0.5200164984937075+1.0975277942502903i, "z (pi/2)"=-1.0311345636926572+0.5736824521422934i, "z center"=-0.5136528600391839+0.580046090596817i, "z(0)"=-0.5200164984937075+1.0975277942502903i, "radius"=-1.0311345636926572} ("circle corners in"), "z center"=w301, "z(0)"=w298) -> (w292:T15)
            n134 = call "peak -- four corner circle transformation logic.vi"("4 corner circle transformation"=four-corner_circle_transformation."z(c) z(zero)", "circle corners in"=w292) -> ("circle corners out"=w297:T15)  [unwired: 8 in, 1 out]
            n135 = call "draw - 4 corner circle.vi"("4corners"=w297) -> ("line two"=→"line two":cluster{dbl[], dbl[]}, "line one"=→"line one":cluster{dbl[], dbl[]}, "circle"=→"circle":cluster{dbl[], dbl[]})  [unwired: 8 in]
          }
          frame "plot all" {
          }
        }
      }
      event "complex plane scale gauge": Value Change {
        n136 = event-data() -> ()  [unwired: 1 in, 1 out]
        n137 = Generate User Event(user event=w308, event data cluster="scale gauge changed" ("event data")) -> ()  [unwired: 1 in, 2 out]
      }
      event "Plot:complex plane": Cursor Move {
        n138 = event-data() -> ()  [unwired: 1 in, 5 out]
        n139 = Generate User Event(user event=w310, event data cluster="draw circle" ("event data")) -> ()  [unwired: 1 in, 2 out]
      }
      event "show plot pallets": Value Change {
        n140 = event-data() -> ("NewVal"=w313:bool)  [unwired: 1 in]
        n141 = property on="Property Node" class="XYGraph (strict)"(reference=w314, "ScaleLegendVis"=w313, "Palette Visible"=w313, "Legend Visible"=w313) -> ()  [unwired: 1 in, 2 out]
        n142 = property on="Property Node" class="XYGraph (strict)"(reference=w312, "ScaleLegendVis"=w313, "Palette Visible"=w313, "Legend Visible"=w313) -> ()  [unwired: 1 in, 2 out]
      }
    }
  }
  n143 = Increment(x=w109) -> (x+1=w105:i32)
  n144 = Divide(x=w105, y=w110) -> (x/y=w113:dbl)
  n145 = Multiply(x=w113, y=100.0) -> (x*y=w111:dbl)
  n146 = local write "Progress, %"(w111) -> ()
  n147 = disable-structure shown="Disabled" {
    frame Disabled {
      n148 = Unbundle By Name() -> ("Lockin mode"=w315:enum16{"SRS", "NI-DAQ"})  [unwired: 1 in]
      n149 = case shown="\"NI-DAQ\"" w315 {
        tunnel: [_ w317] -> _
        tunnel: [_ w316] -> _
        frame "SRS", Default {
        }
        frame "NI-DAQ" {
          # "Download freq array"
          n150 = call "ProgramFreqBulk.vi"() -> ("error out"=w317:errorcluster, "RUS settings out"=w316:T12)  [unwired: 5 in, 5 out]
        }
      }
    }
    frame Enabled {
    }
  }
  n151 = Unbundle By Name("sweep settings") -> ("Zero amplitude\nat the end"=w7:bool, "save freq units"=w6:enum16{"kHz", "Hz"}, "Bypass error dialog"=w8:bool)
  n152 = Array Subset(array=w62, length=w61) -> (w54:dbl[])  [unwired: 1 in]
  n153 = Array Subset(array=w101, length=w61) -> (w71:cdb[])  [unwired: 1 in]
  n154 = call "single sweep - rus clean up.vi"("Zero amplitude at the end"=w7, "Stop user event"=w64, "error in (no error)"=w38, "RUS settings"=w63) -> ("error out"=w95:errorcluster, "STD status byte"=→"STD status byte":u8, "Error status byte\n(bit 5 - FAST aborted)"=→"Error status byte\n(bit 5 - FAST aborted)":u8, "RUS settings out"=w90:T12)  [unwired: 4 in]
  n155 = Complex To Re/Im(x + iy=w71) -> (x=w70:dbl[], y=w69:dbl[])
  n156 = Not(x=w100) -> (.not. x?=w88:bool)
  n157 = disable-structure shown="Enabled" {
    disable-tunnel: w69 -> [w322 w324]
    disable-tunnel: w70 -> [w321 w323]
    disable-tunnel: [w320 w323] -> w67
    disable-tunnel: [w319 w324] -> w66
    disable-tunnel: w98 -> [w318 _]
    frame Disabled {
      n158 = call "Rotate Lockin Phase.vi"("Phase"=w318, "Array Y in"=w322, "Array X in"=w321) -> ("Array Y out"=w319:dbl[], "Array X out"=w320:dbl[])  [unwired: 7 out]
    }
    frame Enabled {
    }
  }
  n159 = case shown="True" w88 {
    tunnel: w95 -> [w325 w332]
    tunnel: [w325 w330] -> w115
    tunnel: w71 -> [_ w327]
    tunnel: w90 -> [_ w329]
    tunnel: w54 -> [_ w328]
    tunnel: w6 -> [_ w326]
    frame False {
    }
    frame True {
      n160 = call "single sweep - save rus data.vi"("save freq units"=w326, "error in (no error)"=w332, "rus response"=w327, "F Array"=w328, "RUS settings"=w329) -> ("error out"=w330:errorcluster, "Actual file path"=→"Actual file path":path)  [unwired: 5 in]
    }
  }
  n161 = Divide(x=w54, y=1000 ("dimension size")) -> (x/y=w53:dbl[])
  n162 = Bundle(w67, w66) -> (w68:cluster{dbl[], dbl[]})  [unwired: 1 out]
  n163 = Bundle(w53, w67) -> (w104:cluster{dbl[], dbl[]})  [unwired: 1 out]
  n164 = Bundle(w53, w66) -> (w103:cluster{dbl[], dbl[]})  [unwired: 1 out]
  n165 = Build Array(w104, w103) -> (w72:cluster{dbl[], dbl[]}[])
  n166 = Build Array(w68) -> (w65:cluster{dbl[], dbl[]}[])
  n167 = disable-structure shown="Disabled" {
    frame Disabled {
      n168 = while {
        shift-right: [w336] -> _
        shift-left: _ -> [w337]
        shift-right: [w335] -> _
        shift-left: _ -> [w338]
        tunnel: [w333] -> _
        stop <- TRUE stop-if-true
        n169 = property class="DAQmx Write"(reference=w337, error in=w338) -> (reference out=w336:refnum<k21>, error out=w335:errorcluster, "SpaceAvail"=w333:u32)
      }
    }
    frame Enabled {
    }
  }
  n170 = local write "Plot:complex plane"(w65) -> ()
  n171 = local write "Plot:response"(w72) -> ()
  n172 = case shown="False" w8 {
    tunnel: [w340 w342] -> w118
    tunnel: w115 -> [w339 w342]
    frame False {
      w341 = T18 3 items=["no dialog", "OK message", "continue or stop message", "OK message + warnings", "continue/stop + warnings"] ("type of dialog (OK msg:1)")
      n173 = call <vilib>:"General Error Handler.vi"("type of dialog (OK msg:1)"=w341, "error in (no error)"=w339) -> ("error out"=w340:errorcluster)  [unwired: 13 out]
    }
    frame True {
    }
  }
  "error out" <- w118
